vi "RequestDestroy.vi"(8 "Error In":errorcluster, 11 "reference in":refnum<class "TraceWindow.lvclass">) -> (0 "Error Out":errorcluster, 3 "reference out":refnum<class "TraceWindow.lvclass">)   [LabVIEW 2021, in "TraceWindow.lvlib" / "TraceWindow.lvclass"]
uses:
  TraceWindow.lvclass
  3fbc1877-3ae8-4aff-a423-cebf9be5a0b1.vi
  MainGUIRepository.vi
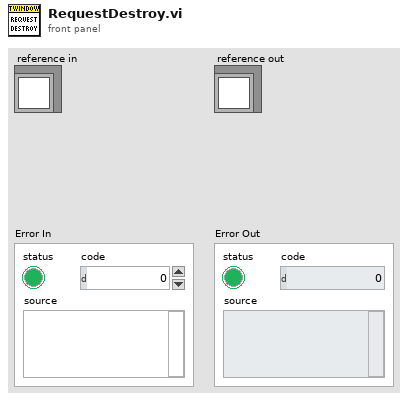
[diagram p1: front panel]
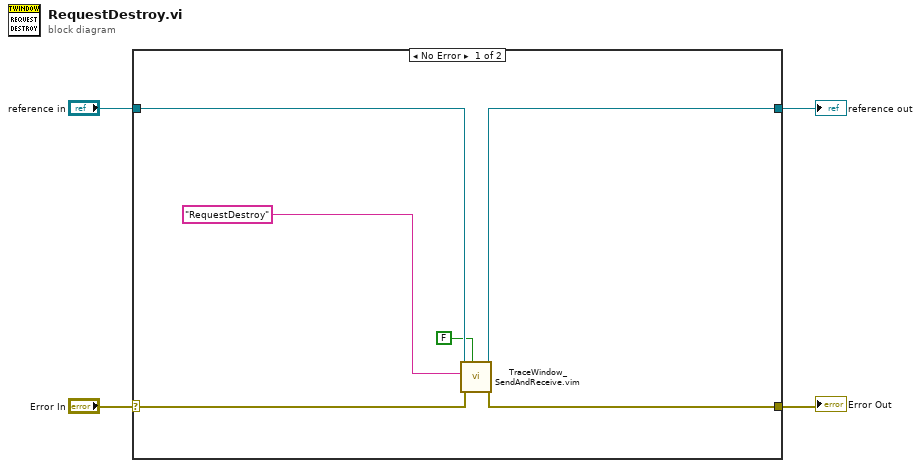
[diagram p0: block diagram]
diagram:
  n1 = case shown="No Error" "Error In" {
    selector: "Error In" -> [w10 w12]
    tunnel: [w9 w12] -> w3
    tunnel: [w7 w11] -> w1
    tunnel: "reference in" -> [w8 w11]
    frame No Error {
      n2 = call "TraceWindow_SendAndReceive.vim"("ShouldWeWaitForResponse"=FALSE, "error in (no error)"=w10, "Command"="RequestDestroy", "reference in"=w8) -> ("error out"=w9:errorcluster, "reference out"=w7:refnum<class "TraceWindow.lvclass">)  [unwired: 5 in, 1 out]
    }
    frame Error {
    }
  }
  "Error Out" <- w3
  "reference out" <- w1
